vi "kf_demodulator.vi"(0 "Reset":bool, 5 "Config":T2={"I/O"={"Format"={"Rate"=4, "Bits"=32, "Channels"=2}, "card #"=1, "# buffers"=96000}, "High rate STFT"={"Win param"=101.5, "Window type"=61, "Win order"=2, "DFT size"=64, "Channels"=[7], "Oversample"=64}, "Low rate STFT"={"Win param"=120.0, "Window type"=61, "Win order"=8, "DFT size"=64, "Channels"=[7], "Oversample"=64}, "Filtering"={"Hum"={"Frequency"=0.0, "Tc"=0.0, "Limit"=101.5, "FFT filter"=FALSE, "Detrend mode"=enum."Robust linear", "Enable"=FALSE}, "Kalman"={"Process noise"=101.5, "Measure noise"=101.5, "Unlock m noise"=101.5, "Mode"=enum."FFT"}, "Distortion"={"LF cut"=101.5, "Tc"=3.0, "Limit"=101.5, "FFT filter"=FALSE, "Detrend mode"=enum."Robust linear", "Enable"=FALSE}, "Lowpass"={"Frequency"=0.0, "Order"=0, "Enable"=FALSE}, "Impulse"={"Win order"=102, "Locked limit"=101.5, "Locked count"=102, "Threshold Tc"=101.5, "Thresh sigmas"=101.5, "Thresh min"=101.5, "After"=0, "Detrend"=FALSE, "Enable"=FALSE}}} {"Filtering"."Impulse"."Thresh min" format="%#_3p"; "Filtering"."Impulse"."Threshold Tc" format="%#_3p"; "Filtering"."Impulse"."Locked limit" format="%#_3p"; "Filtering"."Impulse"."Thresh sigmas" format="%#_3p"; "Filtering"."Lowpass"."Frequency" format="%#_4p"; "Filtering"."Distortion"."Limit" format="%#_3p"; "Filtering"."Distortion"."LF cut" format="%#_3p"; "Filtering"."Kalman"."Unlock m noise" format="%#_3p"; "Filtering"."Kalman"."Measure noise" format="%#_3p"; "Filtering"."Kalman"."Process noise" format="%#_3p"; "Filtering"."Hum"."Limit" format="%#_3p"; "Filtering"."Hum"."Frequency" format="%#_4p"; "Low rate STFT"."Oversample" min=1 step=1; "Low rate STFT"."Channels" min=0 step=1; "Low rate STFT"."DFT size" min=1 step=1; "Low rate STFT"."Window type" items=["Rectangle"=0, "Hanning"=1, "Hamming"=2, "Blackman-Harris"=3, "Exact Blackman"=4, "Blackman"=5, "Flat Top"=6, "4 Term B-Harris "=7, "7 Term B-Harris"=8, "Low Sidelobe"=9, "Blackman Nuttall"=11, "Triangle"=30, "Bartlett-Hanning"=31, "Bohman"=32, "Parzen"=33, "Welch"=34, "Kaiser"=60, "Dolph-Chebyshev"=61, "Gaussian"=62]; "High rate STFT"."Oversample" min=1 step=1; "High rate STFT"."Channels" min=0 step=1; "High rate STFT"."DFT size" min=1 step=1; "High rate STFT"."Window type" items=["Rectangle"=0, "Hanning"=1, "Hamming"=2, "Blackman-Harris"=3, "Exact Blackman"=4, "Blackman"=5, "Flat Top"=6, "4 Term B-Harris "=7, "7 Term B-Harris"=8, "Low Sidelobe"=9, "Blackman Nuttall"=11, "Triangle"=30, "Bartlett-Hanning"=31, "Bohman"=32, "Parzen"=33, "Welch"=34, "Kaiser"=60, "Dolph-Chebyshev"=61, "Gaussian"=62]}, 7 "Modulation info":T8={"Fs full"=0.0, "Fs high"=0.0, "Fs low"=0.0, "Read size"=0, "FFT size low"=5000, "df low"=5000.0, "High carriers"=[], "Low carriers"=[], "Hi channels at low"=[7]} {"Hi channels at low" min=0 step=1; "Low carriers" format="%#_6p"; "High carriers" format="%#_6p"}, 9 "Low carrier amplitudes":cdb[](array[numeric]) format="%#_3p", 11 "Trace info in":T1, 12 "Raw data":dbl[](array[numeric])) -> (4 "Unlocked":bool, 6 "Impulse":bool, 10 "High carrier amplitudes":cdb[][](array[numeric]) format="%_3p", 14 "Filtered signal":dbl[](array[numeric]), 15 "Trace info out":T1)   [LabVIEW 2014]
uses:
  modulation_info.ctl
  ilemt_config.ctl
  io_config.ctl
  stft_params.ctl
  <vilib>/Analysis/4window.llb/windowTd.ctl
  filter_params.ctl
  detrend_mode.ctl
  trace_channel.ctl
  <vilib>/Analysis/NI_AALPro.lvlib
panel:
  out "High carrier amplitudes (iter)":cdb[](array[numeric]) format="%_3p"
  out "Waveform Graph":dbl[][](graph)
  # "This VI deals with high-rate demodulation and filtering for a single sensor axis."
  # "Rows are time (high carrier samples), columns are high rate source XYZ axis amplitudes."
  # "Disabled on block diagram"
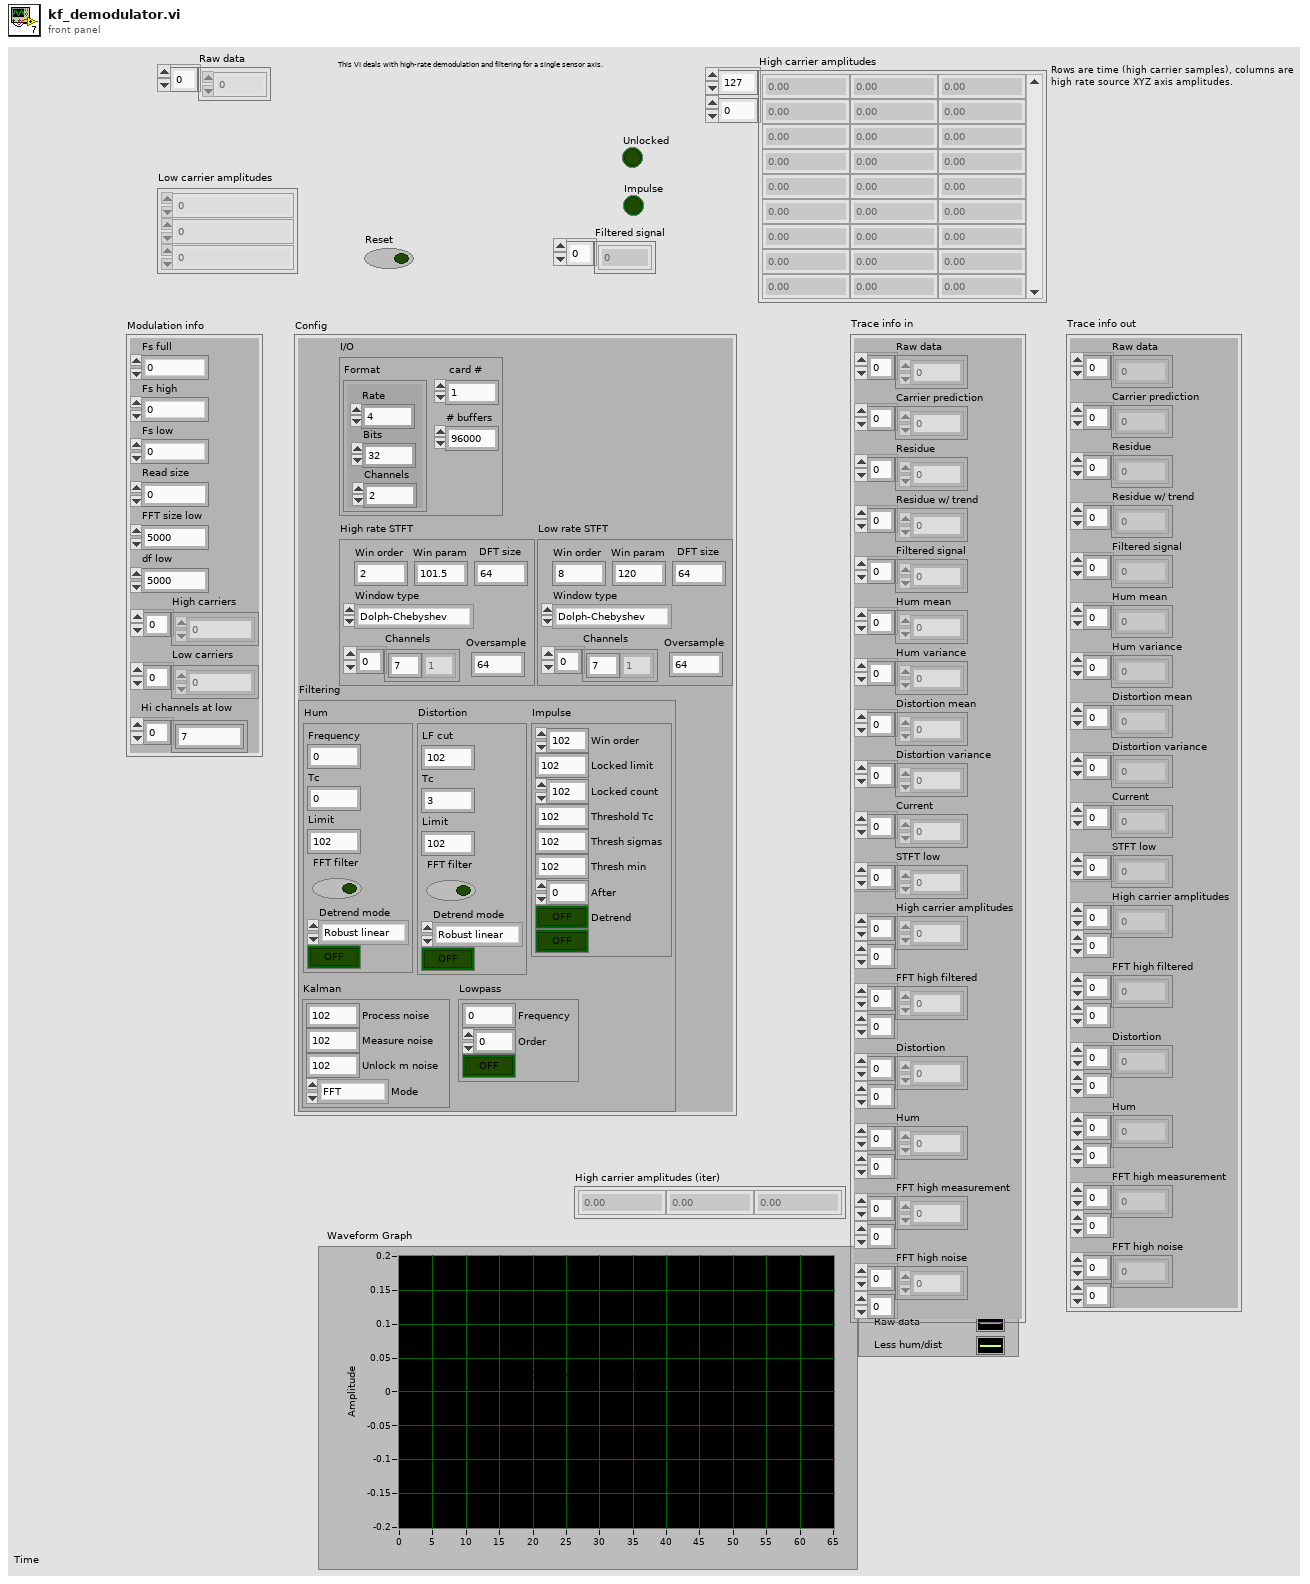
[diagram p1: front panel]
types:
  T1 = typedef "trace_channel.ctl" = cluster{"Raw data":dbl[], "Carrier prediction":dbl[], "Residue":dbl[], "Residue w/ trend":dbl[], "Filtered signal":dbl[], "Hum mean":dbl[], "Hum variance":dbl[], "Distortion mean":dbl[], "Distortion variance":dbl[], "Current":dbl[], "STFT low":cdb[], "High carrier amplitudes":cdb[][], "FFT high filtered":cdb[][], "Distortion":cdb[][], "Hum":cdb[][], "FFT high measurement":cdb[][], "FFT high noise":dbl[][]}
  T2 = typedef "ilemt_config.ctl" = cluster{"I/O":T3, "High rate STFT":T4, "Low rate STFT":T4, "Filtering":T6}
  T3 = typedef "io_config.ctl" = cluster{"Format":cluster{"Rate":i32, "Bits":i32, "Channels":u32}, "card #":u32, "# buffers":i32}
  T4 = typedef "stft_params.ctl" = cluster{"Win param":dbl, "Window type":T5, "Win order":i32, "DFT size":i32, "Channels":i32[], "Oversample":i32}
  T5 = typedef "NI_AALPro.lvlib/windowTd.ctl" = u32
  T6 = typedef "filter_params.ctl" = cluster{"Hum":cluster{"Frequency":dbl, "Tc":dbl, "Limit":dbl, "FFT filter":bool, "Detrend mode":T7, "Enable":bool}, "Kalman":cluster{"Process noise":dbl, "Measure noise":dbl, "Unlock m noise":dbl, "Mode":enum16{"FFT", "KF demod"}}, "Distortion":cluster{"LF cut":dbl, "Tc":dbl, "Limit":dbl, "FFT filter":bool, "Detrend mode":T7, "Enable":bool}, "Lowpass":cluster{"Frequency":dbl, "Order":i32, "Enable":bool}, "Impulse":cluster{"Win order":i32, "Locked limit":dbl, "Locked count":i32, "Threshold Tc":dbl, "Thresh sigmas":dbl, "Thresh min":dbl, "After":i32, "Detrend":bool, "Enable":bool}}
  T7 = typedef "detrend_mode.ctl" = enum16{"Zero mean", "Linear", "Robust linear"}
  T8 = typedef "modulation_info.ctl" = cluster{"Fs full":dbl, "Fs high":dbl, "Fs low":dbl, "Read size":i32, "FFT size low":i32, "df low":dbl, "High carriers":dbl[], "Low carriers":dbl[], "Hi channels at low":i32[]}
  T9 = typedef "averaging_filter_params.ctl" = cluster{"Order":i32, "Time constant":dbl, "Detrend mode":T7, "TD amplitude limit":dbl, "FFT filter":bool, "Notch channels":i32[], "LF cutoff":i32, "FD amplitude limit":dbl}
  T10 = typedef "kalman_filter.ctl" = cluster{"A":T11, "B":T11, "H":T11, "Q":T11, "R":T11, "x":T11, "P":T11, "x lim":dbl[], "y lim":dbl[], "K":T11, "Converge count":i32}
  T11 = typedef "NI_Matrix.lvlib/RealMatrix.ctl" = dbl[][]
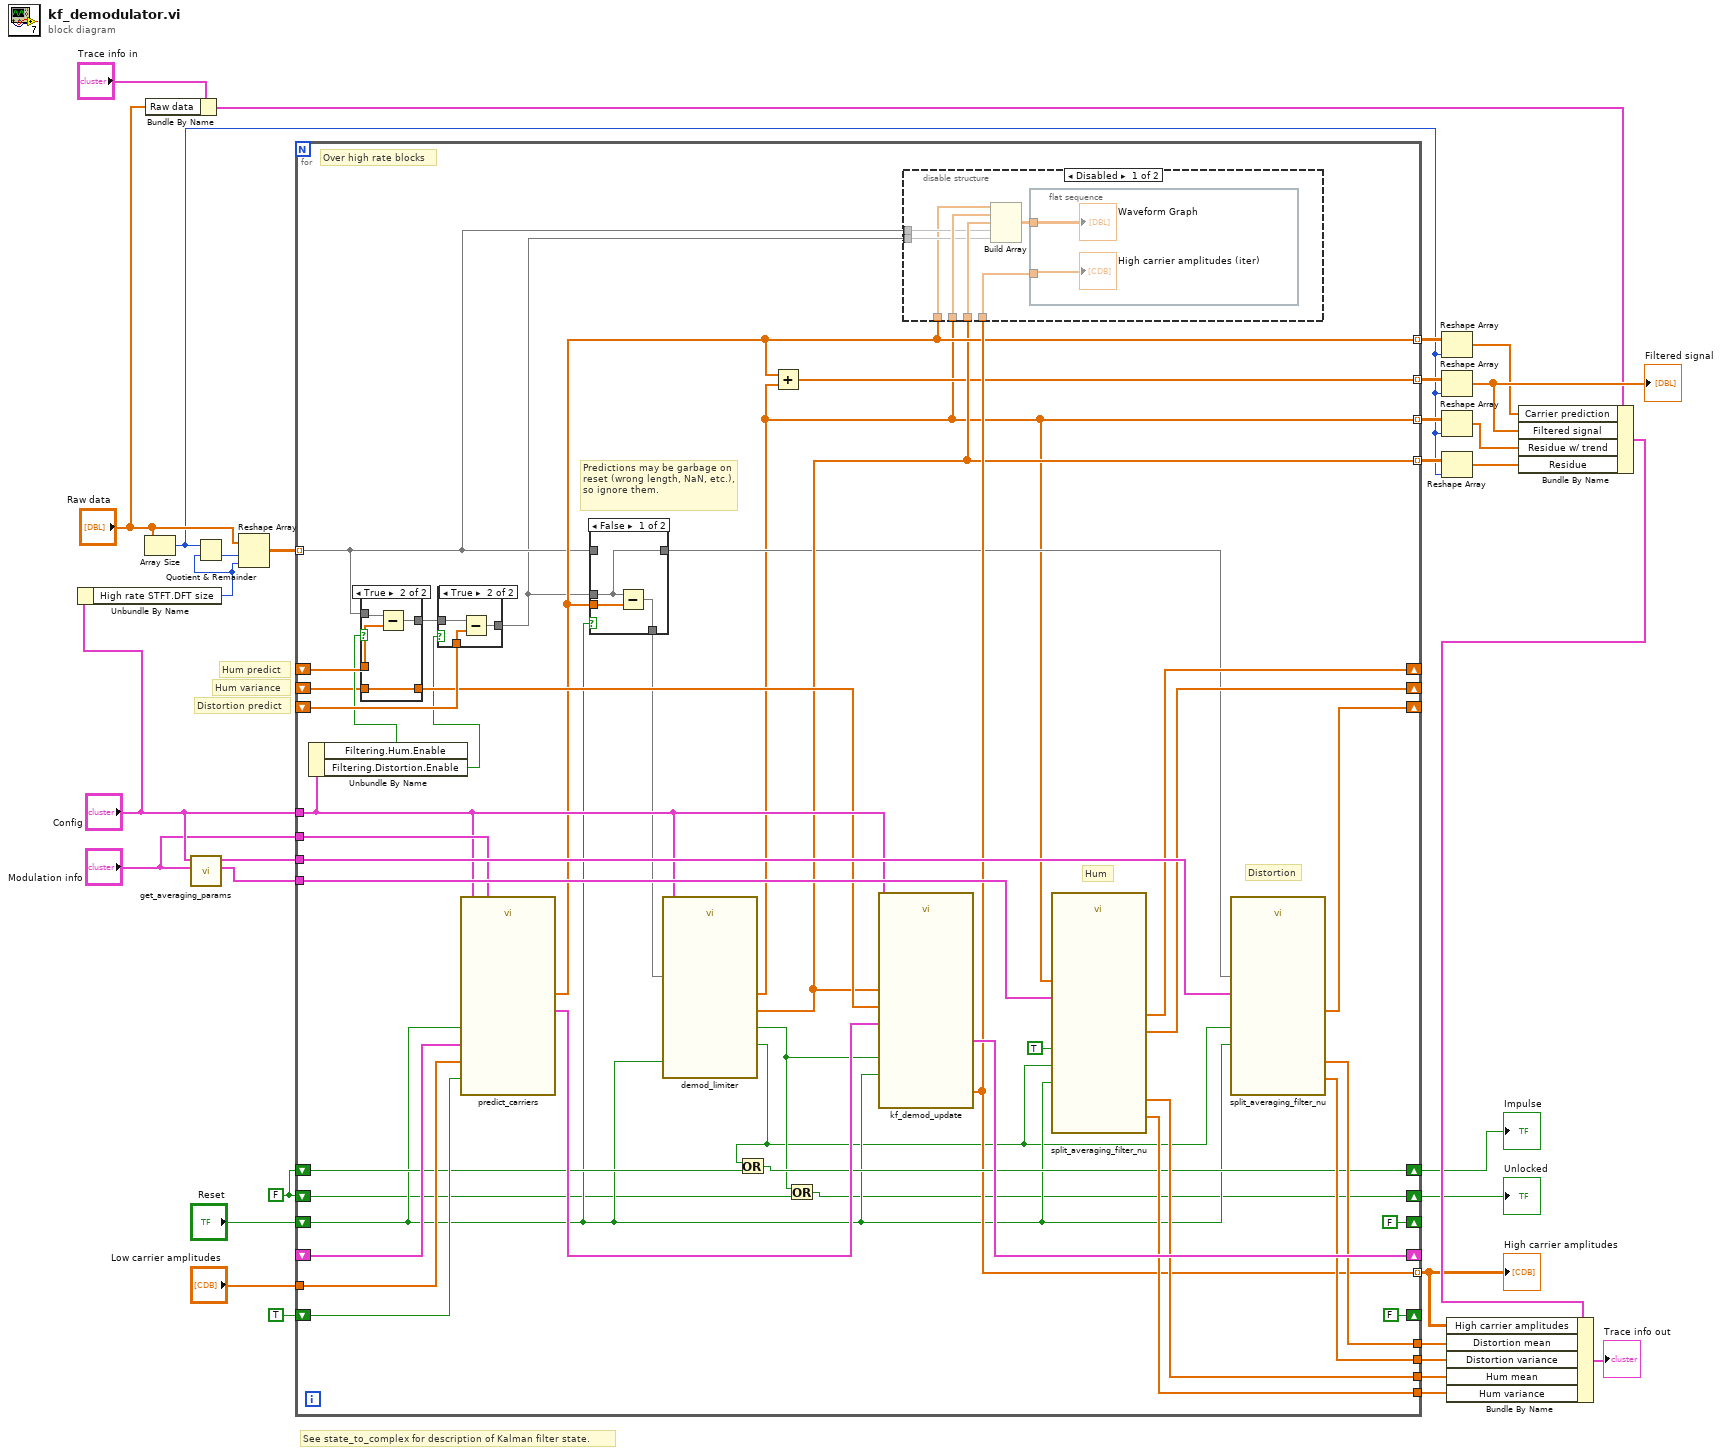
[diagram p0: block diagram]
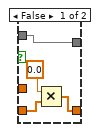
[diagram p5: hidden frame]
diagram:
  w6 = FALSE ("Reset")
  # "Distortion predict"
  # "Hum variance"
  # "Hum predict"
  # "See state_to_complex for description of Kalman filter state."
  n1 = Unbundle By Name("Config") -> ("High rate STFT.DFT size"=w22:i32)
  n2 = Array Size(array="Raw data") -> (size(s)=w3:i32)
  n3 = Bundle By Name(cluster="Trace info in", "Raw data"="Raw data") -> (w10:T1)
  n4 = call "get_averaging_params.vi"("Modulation info"="Modulation info", "Config"="Config") -> ("Hum params"=w30:T9, "Distortion params"=w32:T9)  [unwired: 8 in]
  n5 = Quotient & Remainder(x=w3, y=w22) -> (floor(x/y)=w28:i32)  [unwired: 1 out]
  n6 = Reshape Array("Raw data", w28, w22) -> (w29:dbl[][])
  n7 = for {
    tunnel: w32 -> [w72]
    tunnel: w29 -> [w45] mode=indexing
    tunnel: w30 -> [w71]
    shift-right: [FALSE ("Reset")] -> _
    shift-left: "Reset" -> [w42]
    shift-right: [w68] -> _
    shift-left: _ -> [w70]
    tunnel: "Config" -> [w54]
    tunnel: "Low carrier amplitudes" -> [w69]
    tunnel: [w47] -> w1 mode=indexing
    shift-right: [w67] -> _
    shift-left: _ -> [w64]
    shift-right: [w66] -> _
    shift-left: _ -> [w52]
    shift-right: [w65] -> _
    shift-left: _ -> [w63]
    shift-right: [FALSE ("Reset")] -> _
    shift-left: TRUE ("Reset") -> [w60]
    tunnel: "Modulation info" -> [w59]
    tunnel: [w58] -> w19
    tunnel: [w57] -> w18
    tunnel: [w56] -> w17
    tunnel: [w55] -> w16
    tunnel: [w41] -> w23 mode=indexing
    tunnel: [w40] -> w14 mode=indexing
    shift-right: [w34] -> w9
    shift-left: w6 -> [w38]
    tunnel: [w36] -> w8 mode=indexing
    shift-right: [w49] -> w5
    shift-left: w6 -> [w50]
    tunnel: [w46] -> w4 mode=indexing
    # "Over high rate blocks"
    # "Predictions may be garbage on reset (wrong length, NaN, etc.), so ignore them."
    # "Distortion"
    # "Hum"
    n8 = Unbundle By Name(w54) -> ("Filtering.Hum.Enable"=w53:bool, "Filtering.Distortion.Enable"=w48:bool)
    n9 = case shown="True" w53 {
      tunnel: [w95 w99] -> w73
      tunnel: w64 -> [_ w98]
      tunnel: w45 -> [w95 w97]
      tunnel: w52 -> [w94 w96]
      tunnel: [w93 w96] -> w51
      frame False {
        n10 = Multiply(x=0.0, y=w94) -> (x*y=w93:dbl[])
      }
      frame True {
        n11 = Subtract(x=w97, y=w98) -> (x-y=w99:dbl[])
      }
    }
    n12 = case shown="True" w48 {
      tunnel: w73 -> [w88 w91]
      tunnel: w63 -> [_ w90]
      tunnel: [w88 w89] -> w43
      frame False {
      }
      frame True {
        n13 = Subtract(x=w91, y=w90) -> (x-y=w89:dbl[])
      }
    }
    n14 = call "predict_carriers.vi"("Modulation info"=w59, "Low rate block start"=w60, "Low carrier amplitudes"=w69, "KF in"=w70, "Reset"=w42, "Config"=w54) -> ("KF out"=w62:T10, "Predicted carriers"=w46:dbl[])  [unwired: 4 in]
    n15 = case shown="False" w42 {
      tunnel: w46 -> [w77 _]
      tunnel: w43 -> [w75 _]
      tunnel: w45 -> [_ w78]
      tunnel: [w76 w78] -> w44
      tunnel: [w75 w78] -> w37
      frame False {
        n16 = Subtract(x=w75, y=w77) -> (x-y=w76:dbl[])
      }
      frame True {
      }
    }
    n17 = call "demod_limiter.vi"("Reset"=w42, "Config"=w54, "Residue in"=w44) -> ("Impulse"=w33:bool, "Unlocked"=w35:bool, "Residue w/ trend"=w36:dbl[], "Residue out"=w41:dbl[])  [unwired: 5 in]
    n18 = Or(x=w33, y=w50) -> (x .or. y?=w49:bool)
    n19 = Add(x=w46, y=w36) -> (x+y=w40:dbl[])
    n20 = Or(x=w35, y=w38) -> (x .or. y?=w34:bool)
    n21 = call "kf_demod_update.vi"("Unlocked"=w35, "Reset"=w42, "Variance"=w51, "KF in"=w62, "Config"=w54, "Error"=w41) -> ("KF out"=w68:T10, "New amplitudes"=w47:cdb[])  [unwired: 4 in]
    n22 = disable-structure shown="Disabled" {
      disable-tunnel: w36 -> [w84 _]
      disable-tunnel: w41 -> [w83 _]
      disable-tunnel: w45 -> [w82 _]
      disable-tunnel: w43 -> [w81 _]
      disable-tunnel: w47 -> [w80 _]
      disable-tunnel: w46 -> [w79 _]
      frame Disabled {
        n23 = Build Array(w79, w84, w83, w82, w81) -> (w85:dbl[][])
        n24 = flat-sequence {
          tunnel: w85 -> [w87]
          tunnel: w80 -> [w86]
          frame #0 {
            "Waveform Graph" <- w87
            "High carrier amplitudes (iter)" <- w86
          }
        }
      }
      frame Enabled {
      }
    }
    n25 = call "split_averaging_filter_nu.vi"("Reset"=w42, "Parameters"=w71, "Noise"=w33, "Error mode"=TRUE, "Signal"=w36) -> ("Order variance"=w55:dbl[], "Order mean"=w56:dbl[], "Variance"=w66:dbl[], "Prediction"=w67:dbl[])  [unwired: 3 in]
    n26 = call "split_averaging_filter_nu.vi"("Reset"=w42, "Parameters"=w72, "Noise"=w33, "Signal"=w37) -> ("Order variance"=w57:dbl[], "Order mean"=w58:dbl[], "Prediction"=w65:dbl[])  [unwired: 4 in, 1 out]
  }
  "High carrier amplitudes" <- w1
  "Unlocked" <- w9
  "Impulse" <- w5
  n27 = Reshape Array(w4, w3) -> (w2:dbl[])
  n28 = Reshape Array(w14, w3) -> (w13:dbl[])
  "Filtered signal" <- w13
  n29 = Reshape Array(w8, w3) -> (w7:dbl[])
  n30 = Reshape Array(w23, w3) -> (w21:dbl[])
  n31 = Bundle By Name(cluster=w10, "Carrier prediction"=w2, "Filtered signal"=w13, "Residue w/ trend"=w7, "Residue"=w21) -> (w20:T1)
  n32 = Bundle By Name(cluster=w20, "High carrier amplitudes"=w1, "Distortion mean"=w19, "Distortion variance"=w18, "Hum mean"=w17, "Hum variance"=w16) -> (→"Trace info out":T1)
